vi "GetRingType.vi"(8 "error in (no error)":errorcluster, 11 "Control Ref In":refnum<vi>) -> (0 "error out":errorcluster, 2 "Ring Type":string, 3 "Control Ref Out":refnum<vi>)   [LabVIEW 2014]
panel:
  in  "Ring Types":string[][](array[string])=[["21601", "Text Ring"], ["21600", "Menu Ring"], ["21605", "Enum"], ["21602", "Pict Ring"], ["21603", "Text & Pict Ring"]]
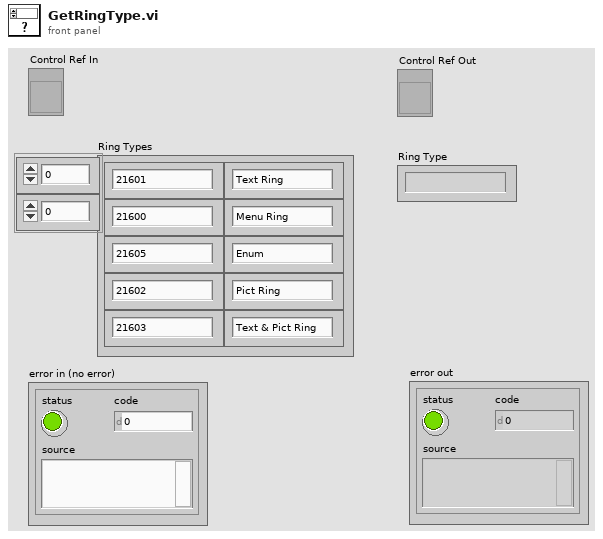
[diagram p1: front panel]
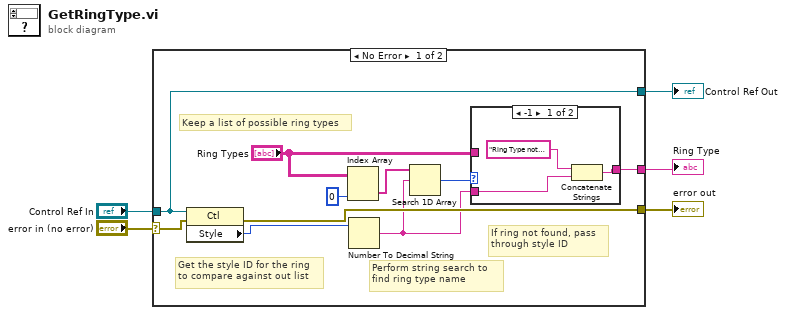
[diagram p0: block diagram]
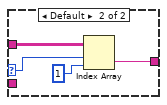
[diagram p2: hidden frame]
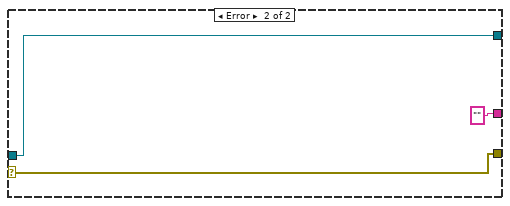
[diagram p3: hidden frame]
diagram:
  n1 = case shown="No Error" "error in (no error)" {
    selector: "error in (no error)" -> [w11 w25]
    tunnel: [w15 w25] -> w5
    tunnel: "Control Ref In" -> [w6 w23]
    tunnel: [w7 "" ("String")] -> w3
    tunnel: [w6 w23] -> w1
    frame No Error {
      # "If ring not found, pass\nthrough style ID"
      # "Perform string search to \nfind ring type name"
      # "Get the style ID for the ring \nto compare against out list"
      # "Keep a list of possible ring types"
      n2 = property class="Ctl"(reference=w6, error in=w11) -> (error out=w15:errorcluster, "Style"=w12:u32)  [unwired: 1 out]
      n3 = Index Array(array="Ring Types", index (col)=0 ("disabled index (col)")) -> (element=w13:string[])  [unwired: 1 in]
      n4 = Number To Decimal String(number=w12) -> (decimal integer string=w9:string)  [unwired: 1 in]
      n5 = Search 1D Array(1D array=w13, element=w9) -> (index of element=w10:i32)  [unwired: 1 in]
      n6 = case shown="-1" w10 {
        selector: w10 -> [_ w19]
        tunnel: "Ring Types" -> [_ w21]
        tunnel: [w17 w20] -> w7
        tunnel: w9 -> [w16 _]
        frame -1 {
          n7 = Concatenate Strings("Ring Type not found: " ("String"), w16) -> (w17:string)
        }
        frame Default {
          n8 = Index Array(array=w21, index (row)=w19, index (col)=1) -> (element=w20:string)
        }
      }
    }
    frame Error {
    }
  }
  "error out" <- w5
  "Ring Type" <- w3
  "Control Ref Out" <- w1
